vi "loopproperties.vi"() -> ()   [LabVIEW 2019]
uses:
  <vilib>/Math Plots/3D Math Plots/3D Surface/3D Surface XCtrl/3D Surface.xctl
  <vilib>/Math Plots/3D Math Plots/3D Surface/3D Surface Datatype/Public/Plot Helper (Vector).vi
  <vilib>/Math Plots/3D Math Plots/3D Surface/3D Surface Datatype/3D Surface Datatype.lvclass
panel:
  out "3D Surface":refnum<class "3D Plot Datatype.lvclass">[](xcontrol)
  out "Array 5":i32[][](array[numeric])
  out "Array 4":i32[][](array[numeric])
  out "out":i8
  out "in":i8
  out "Array 3":string[](array[string])
  out "String":string
  out "Array 2":i8[][](array[numeric])
  out "Numeric 7":i8
  out "Array":i8[](array[numeric])
  in  "Numeric 6":i16
  out "Numeric 5":i32
  in  "Numeric 4":i16
  in  "Numeric 3":i16
  out "x or y":i16
  out "x .and. y?":i16
  in  "Numeric 2":i16
  in  "Numeric":i16
  out "x+y 4":i32[](array[numeric])
  out "x+y 3":i32[](array[numeric])
  out "x+y 2":i32[](array[numeric])
  out "x+y":dbl
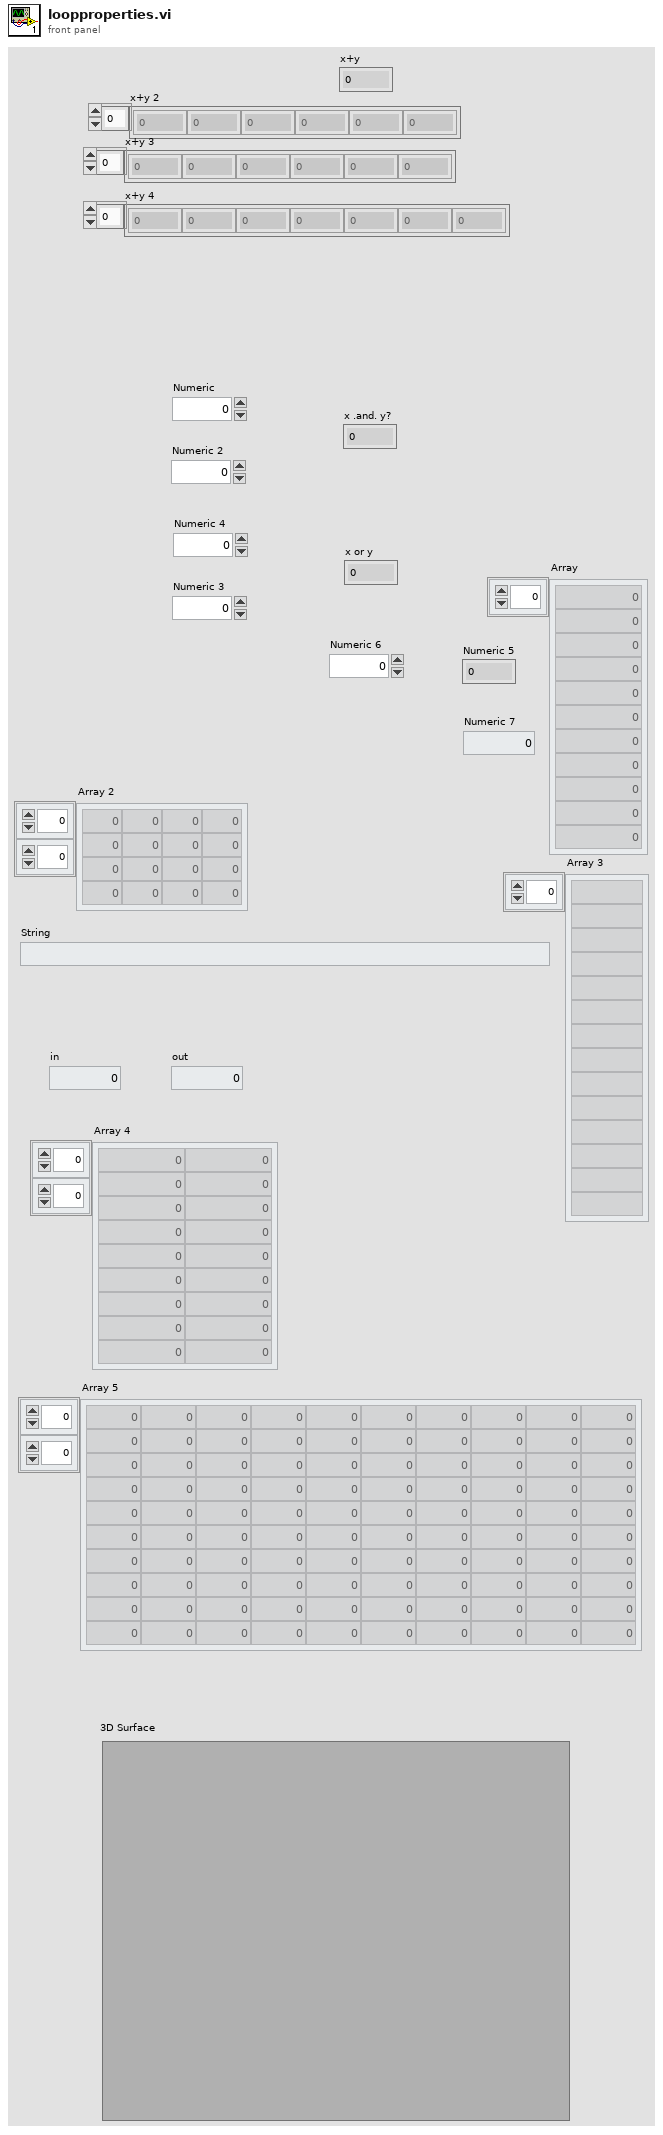
[diagram p1: front panel]
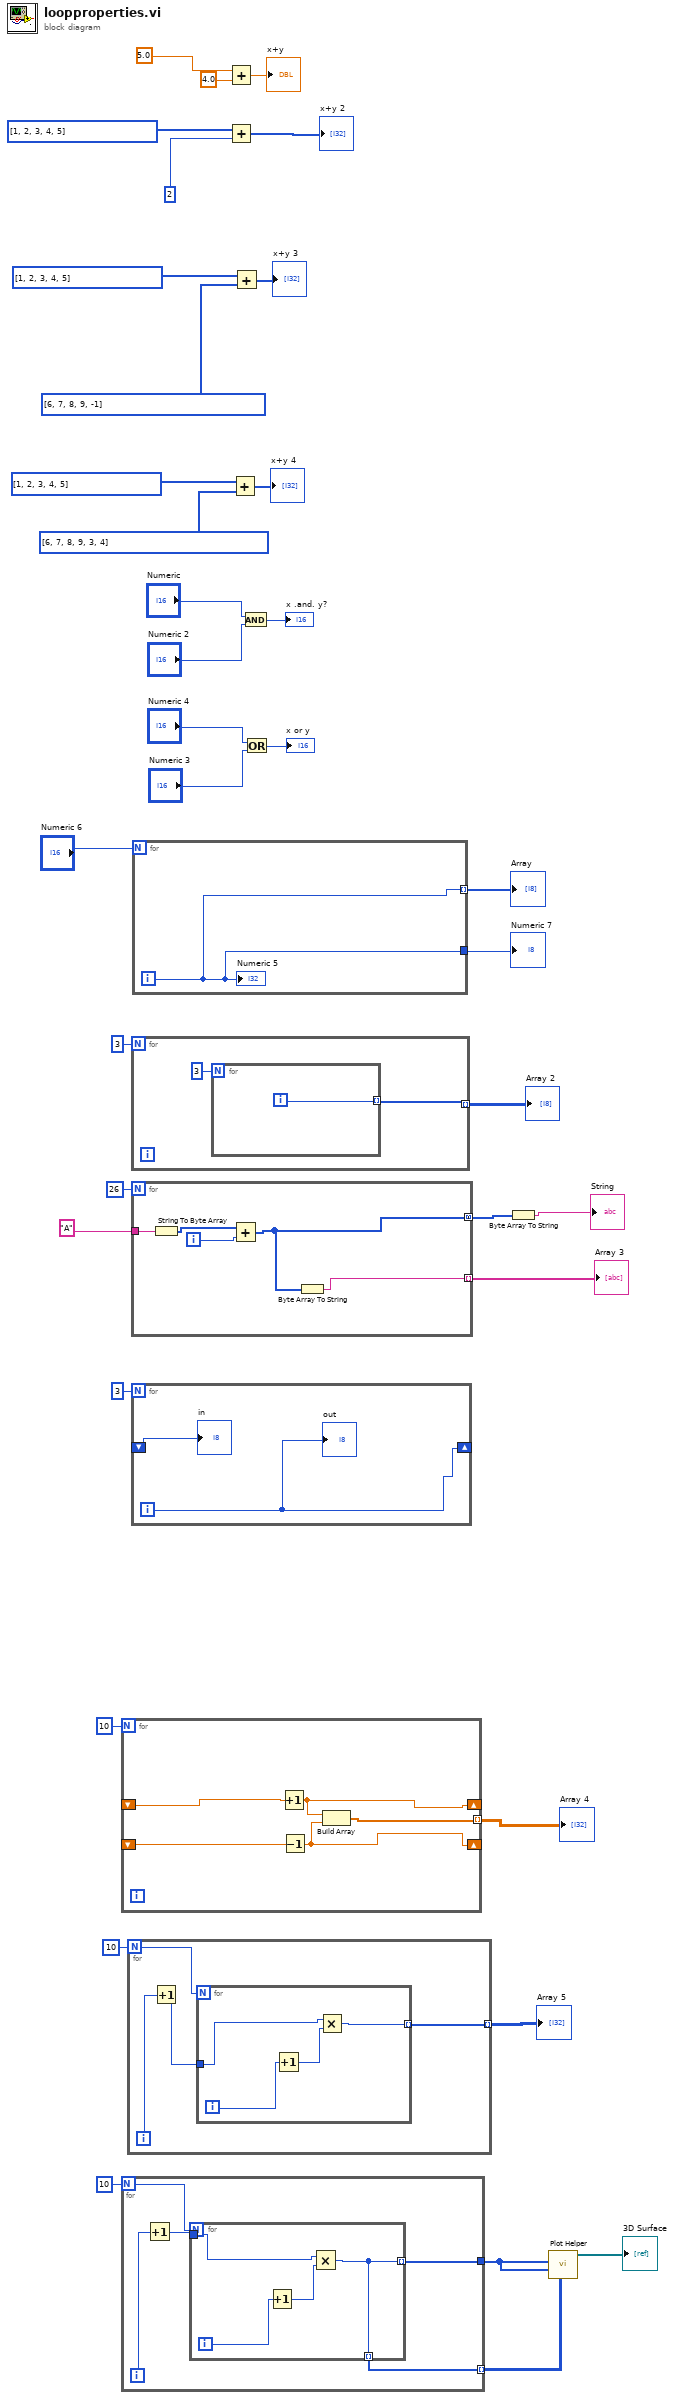
[diagram p0: block diagram]
diagram:
  n1 = for {
    N: 10 -> [_]
    shift-right: [w40] -> _
    shift-left: _ -> [w42]
    shift-right: [w39] -> _
    shift-left: _ -> [w41]
    tunnel: [w38] -> w8 mode=indexing
    n2 = Increment(x=w42) -> (x+1=w40:dbl)
    n3 = Decrement(x=w41) -> (x-1=w39:dbl)
    n4 = Build Array(w40, w39) -> (w38:dbl[])
  }
  "Array 4" <- w8
  n5 = for {
    N: 10 -> [w45]
    tunnel: [w44] -> w1
    tunnel: [w43] -> w2 mode=indexing
    i -> [w47]
    n6 = Increment(x=w47) -> (x+1=w46:i32)
    n7 = for {
      N: w45 -> [_]
      tunnel: w46 -> [w49]
      tunnel: [w48] -> w44 mode=indexing
      tunnel: [w48] -> w43 mode=indexing
      i -> [w51]
      n8 = Increment(x=w51) -> (x+1=w50:i32)
      n9 = Multiply(x=w49, y=w50) -> (x*y=w48:i32)
    }
  }
  n10 = for {
    N: 10 -> [w54]
    tunnel: [w53] -> w5 mode=indexing
    i -> [w55]
    n11 = Increment(x=w55) -> (x+1=w52:i32)
    n12 = for {
      N: w54 -> [_]
      tunnel: w52 -> [w57]
      tunnel: [w56] -> w53 mode=indexing
      i -> [w59]
      n13 = Increment(x=w59) -> (x+1=w58:i32)
      n14 = Multiply(x=w57, y=w58) -> (x*y=w56:i32)
    }
  }
  "Array 5" <- w5
  n15 = for {
    N: 3 -> [_]
    tunnel: [w60] -> w15 mode=indexing
    n16 = for {
      N: 3 -> [_]
      tunnel: [w62] -> w60 mode=indexing
      i -> [w62]
    }
  }
  "Array 2" <- w15
  n17 = for {
    N: 26 -> [_]
    tunnel: "A" -> [w67]
    tunnel: [w64] -> w12 mode=concatenating
    tunnel: [w63] -> w10 mode=indexing
    i -> [w65]
    n18 = String To Byte Array(string=w67) -> (unsigned byte array=w66:u8[])
    n19 = Add(x=w66, y=w65) -> (x+y=w64:i32[])
    n20 = Byte Array To String(unsigned byte array=w64) -> (string=w63:string)
  }
  "Array 3" <- w10
  n21 = for {
    N: 3 -> [_]
    shift-right: [w68] -> _
    shift-left: _ -> [w69]
    i -> [w68]
    "in" <- w69
    "out" <- w68
  }
  n22 = for {
    N: "Numeric 6" -> [_]
    tunnel: [w70] -> w18 mode=indexing
    tunnel: [w70] -> w17
    i -> [w70]
    "Numeric 5" <- w70
  }
  "Array" <- w18
  "Numeric 7" <- w17
  n23 = Add(x=5.0, y=4.0) -> (x+y=→"x+y":dbl)
  n24 = Add(x=i32[] [1, 2, 3, 4, 5], y=2) -> (x+y=→"x+y 2":i32[])
  n25 = Add(x=i32[] [1, 2, 3, 4, 5], y=i32[] [6, 7, 8, 9, 3, 4]) -> (x+y=→"x+y 4":i32[])
  n26 = Add(x=i32[] [1, 2, 3, 4, 5], y=i32[] [6, 7, 8, 9, -1]) -> (x+y=→"x+y 3":i32[])
  n27 = And(x="Numeric", y="Numeric 2") -> (x .and. y?=→"x .and. y?":i16)
  n28 = Or(x="Numeric 4", y="Numeric 3") -> (x .or. y?=→"x or y":i16)
  n29 = Byte Array To String(unsigned byte array=w12) -> (string=→"String":string)
  n30 = call-poly <vilib>:"Plot Helper.vi"("z matrix"=w2, "y vector"=w1, "x vector"=w1) -> ("3D Plot lvclass Array out"=→"3D Surface":refnum<class "3D Plot Datatype.lvclass">[])  [unwired: 3 in, 5 out]
